vi "Add Actions to Stack.vi"(7 "Add to top of Stack":string, 11 "Action Stack":string) -> (3 "Action Stack out":string)   [LabVIEW 2020, in "Action Stack.lvlib"]
doc: "Add one or more actions to the top of the Stack.\n\n<B>Action Syntax:</B>\nAction >> Argument\nAction separator: Line feed\nTo add a comment use \"//\" or \"#\" and all text to the right will be ignored\n\n<B>Example:</B>\n//Initial Actions\nUI:Initialize // This initializes the UI\nData:Initialize\nUpdate >> Full // initial update of everything"
uses:
  <vilib>/JDP Science/JDP Science Common Utilities/Action Stack/Action Stack.lvlib
  <vilib>/JDP Science/JDP Science Common Utilities/JDP Utility.lvlib
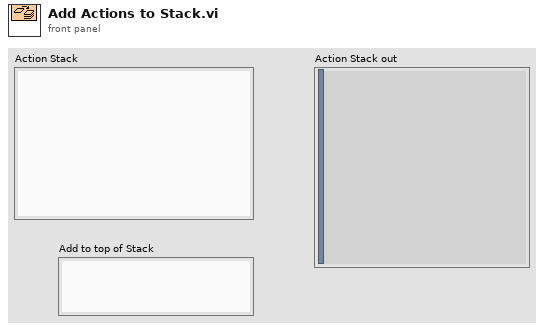
[diagram p1: front panel]
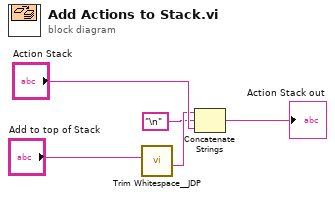
[diagram p0: block diagram]
diagram:
  n1 = call <vilib>:"Trim Whitespace__JDP.vi"("String in"="Add to top of Stack") -> ("String out"=w2:string)  [unwired: 6 in]
  n2 = Concatenate Strings(w2, "\n" ("string"), "Action Stack") -> (→"Action Stack out":string)
